vi "Render Comment.vi"(8 "Error In":errorcluster) -> (0 "Error Out":errorcluster)   [LabVIEW 2018, in "Tests.lvlib" / "Render.lvlib"]
uses:
  Render.lvlib
  <vilib>/addons/_JKI Toolkits/Caraya/classes/Test/Test.lvclass
  <vilib>/addons/_JKI Toolkits/Caraya/classes/Assert/Assert.lvclass
  src/Toolkit/Low-Level/Support/Lex String.vi
  src/Toolkit/Data/Null/Null.lvclass
  src/Toolkit/Low-Level/Renderer/Abstract/Render to String.vi
  src/Toolkit/Low-Level/Compiler/Compiler.lvclass
  D:/Users/cfield/Code/Field R&D Services/Labstache/src/Toolkit/Data/Datum/Datum.lvclass
  src/Toolkit/Low-Level/Nodes/Root/Root.lvclass
  D:/Users/cfield/Code/Field R&D Services/Labstache/src/Toolkit/Low-Level/Nodes/NonTerminal/NonTerminal.lvclass
  D:/Users/cfield/Code/Field R&D Services/Labstache/src/Toolkit/Low-Level/Nodes/Node/Node.lvclass
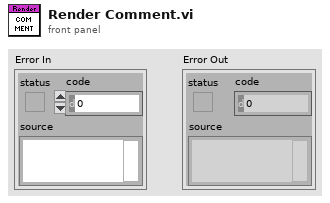
[diagram p1: front panel]
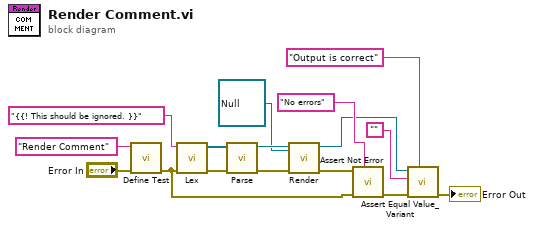
[diagram p0: block diagram]
diagram:
  n1 = call <vilib>:"Define Test.vi"("error in (no error)"="Error In", "Label (VI Title)"="Render Comment") -> ("error out"=w5:errorcluster)  [unwired: 9 in]
  n2 = call-poly "Lex.vi"("Error In"=w5, "Input"="{{! This should be ignored. }}") -> ("Error Out"=w6:errorcluster, "Tokens"=w7:refnum<class "Token.lvclass">[])  [unwired: 8 in]
  n3 = call "Parse.vi"("Error In"=w6, "Tokens"=w7) -> ("Error Out"=w8:errorcluster, "Abstract Syntax Tree"=w4:refnum<class "Root.lvclass">)  [unwired: 8 in]
  n4 = call-poly "Render.vi"(7:refnum<class "Null.lvclass"> refnum ("Toolkit.lvlib:Data.lvlib:Null.lvclass"), "Error In"=w8, "Context In"=w4) -> ("Error Out"=w10:errorcluster, "Context Out"=w9:refnum<class "Compiler.lvclass">)  [unwired: 6 in, 1 out]
  n5 = call <vilib>:"Assert Not Error.vi"("Label"="No errors", "error in (no error)"=w5, "Not Error?"=w10) -> ("error out"=w13:errorcluster)  [unwired: 8 in]
  n6 = call <vilib>:"Assert Equal Value_Variant.vi"("Label"="Output is correct", "error in (no error)"=w13, "Y"="", "X"=w9) -> ("error out"=→"Error Out":errorcluster)  [unwired: 7 in]
